vi "command_TCU.vi"(8 "error in (no error)":errorcluster, 9 "baud rate (115200)":u32=115200, 10 "COM port":refnum<visa-resource-name>="COM4", 11 "Serial_command":string) -> (0 "error out":errorcluster)   [LabVIEW 2018]
uses:
  SupportVIs/VISA Configure Serial Port (Instr).vi
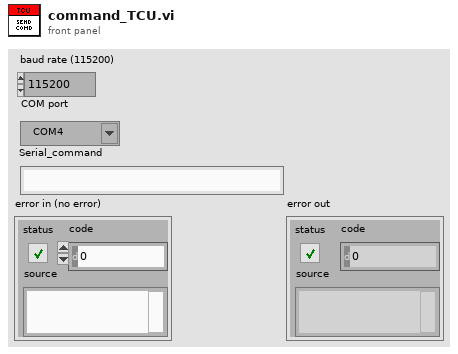
[diagram p1: front panel]
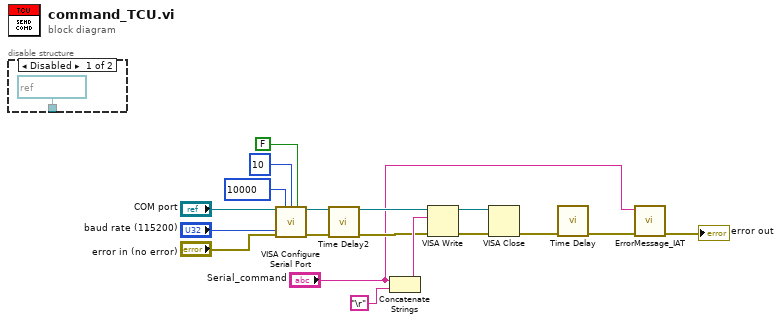
[diagram p0: block diagram]
diagram:
  n1 = disable-structure shown="Disabled" {
    disable-tunnel: [refnum<visa-resource-name> "COM3" ("VISA resource name") _] -> _
    frame Disabled {
    }
    frame Enabled {
    }
  }
  n2 = call-poly "VISA Configure Serial Port"("VISA resource name"="COM port", "timeout (10sec)"=u32 10000, "termination char\n(0xA = '\\n' = LF)"=u8 10 ("termination char\n(0xA = '\\n' = LF)"), "Enable Termination\nChar (T)"=FALSE ("Enable Termination\nChar (T)"), "baud rate (9600)"="baud rate (115200)", "error in (no error)"="error in (no error)") -> ("VISA resource name out"=w7:refnum<visa-resource-name>, "error out"=w9:errorcluster)  [unwired: 8 in]
  n3 = call "Time Delay2"("error in (no error)"=w9) -> ("error out"=w8:errorcluster)  [unwired: 10 in]
  n4 = Concatenate Strings("Serial_command", "\r") -> (w14:string)
  n5 = VISA Write(VISA resource name=w7, write buffer=w14, error in (no error)=w8) -> (VISA resource name out=w12:refnum<visa-resource-name>, error out=w11:errorcluster)  [unwired: 1 out]
  n6 = VISA Close(VISA resource name=w12, error in (no error)=w11) -> (error out=w10:errorcluster)
  n7 = call "Time Delay"("error in (no error)"=w10) -> ("error out"=w3:errorcluster)  [unwired: 10 in]
  n8 = call "ErrorMessage_IAT.vi"("error in (no error)"=w3, "Message"="Serial_command") -> ("error out"=→"error out":errorcluster)  [unwired: 9 in]
